vi "Analisis de fotos con video al tiempo.vi"() -> ()   [LabVIEW 2017]
uses:
  <vilib>/userdefined/High Color/IMAQdx.ctl
  <vilib>/vision/driver/NI_Vision_Acquisition_Software.lvlib
panel:
  in  "Puerto camara":T1
  in  "stop":bool
  out "Video":T2(plugin-control)
  in  "OK Button":bool
  out "Reconocimiento 2":T2(plugin-control)
  out "String (OCR/OCV 2\n)":string
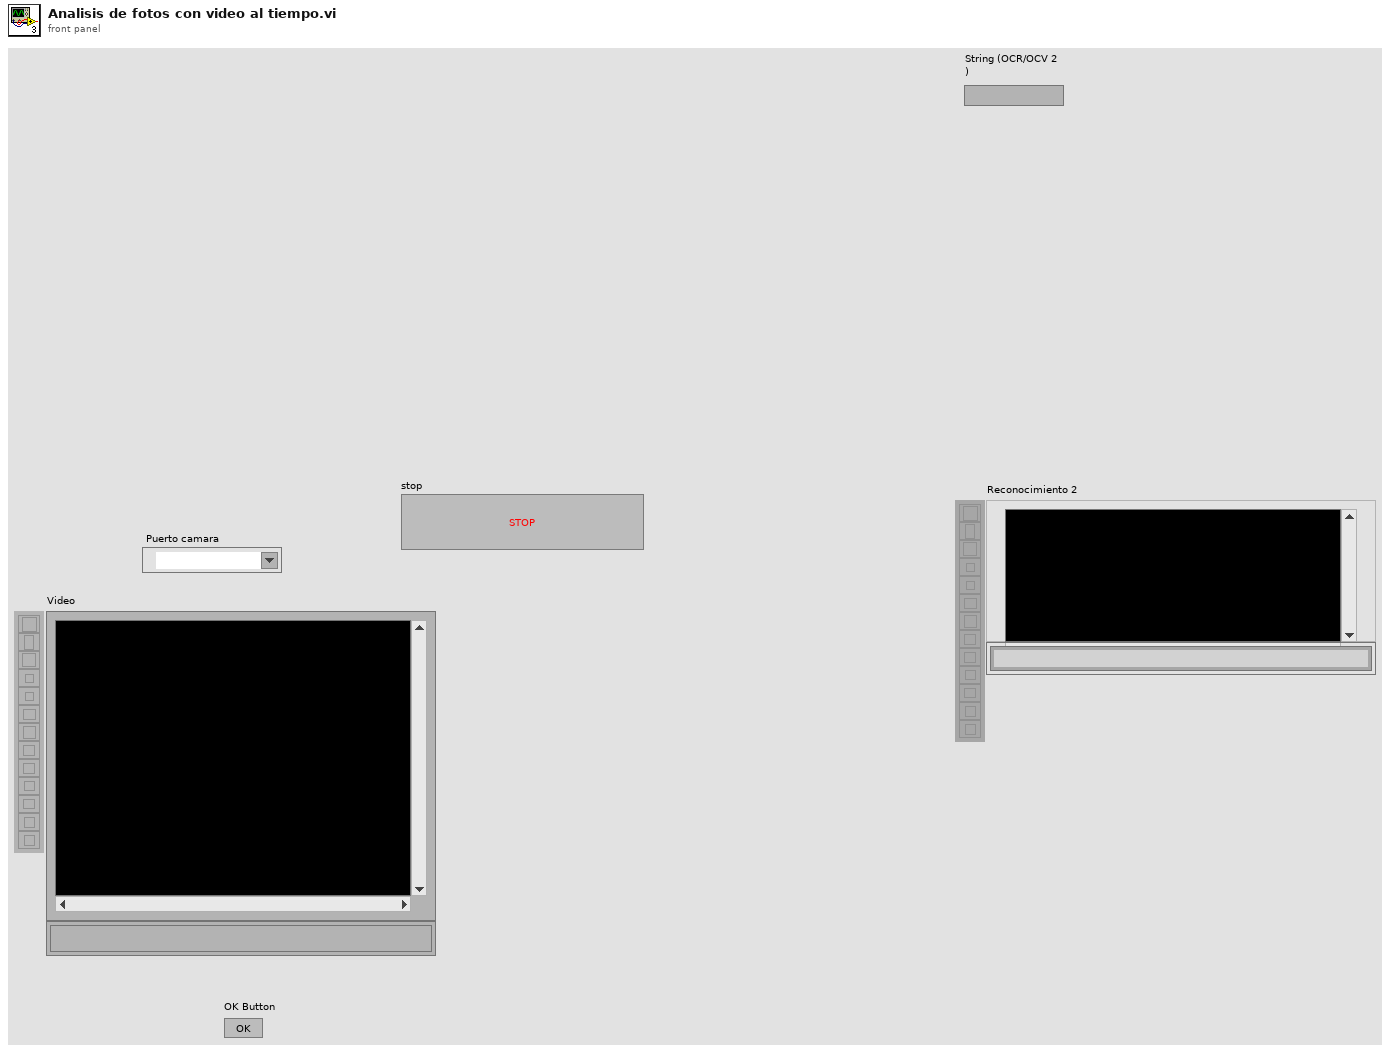
[diagram p1: front panel]
types:
  T1 = typedef "IMAQdx.ctl" = refnum<k21>
  T2 = typedef "IMAQ Image.ctl" = refnum<image>
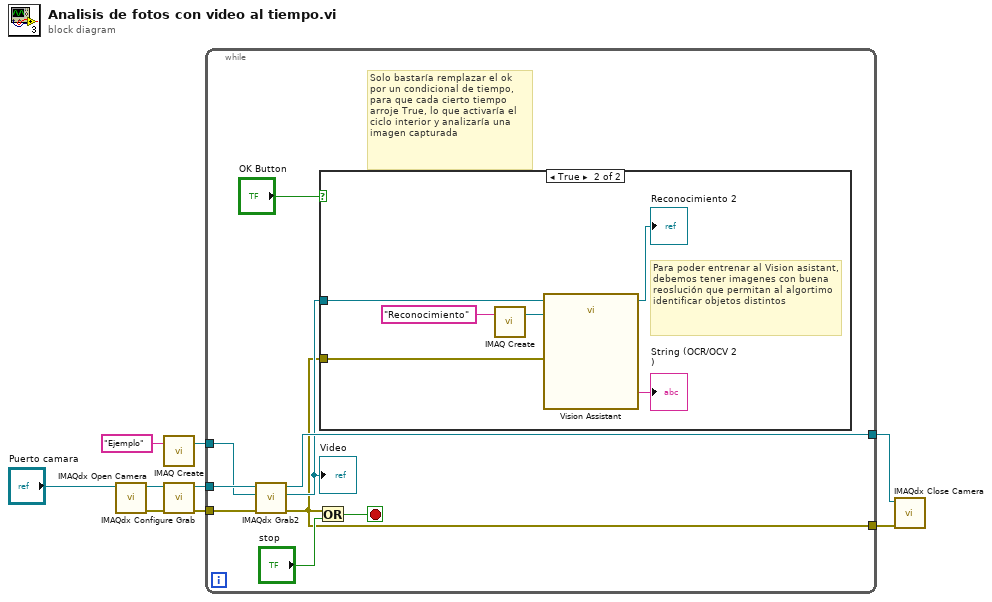
[diagram p0: block diagram]
diagram:
  n1 = call <vilib>:"IMAQdx Open Camera.vi"("Session In"="Puerto camara") -> ("error out"=w4:errorcluster, "Session Out"=w5:T1)  [unwired: 9 in]
  n2 = call "IMAQ Create"("Image Name"="Ejemplo") -> ("New Image"=w1:T2)  [unwired: 4 in, 1 out]
  n3 = call <vilib>:"IMAQdx Configure Grab.vi"("error in"=w4, "Session In"=w5) -> ("error out"=w3:errorcluster, "Session Out"=w6:T1)  [unwired: 8 in]
  n4 = while {
    tunnel: [w18] -> w7
    tunnel: w6 -> [w17]
    tunnel: w3 -> [w16]
    tunnel: [w11] -> w2
    tunnel: w1 -> [w15]
    stop <- w13 stop-if-true
    # "Solo bastaría remplazar el ok por un condicional de tiempo, para que cada cierto tiempo arroje True, lo que activaría el  ciclo interior y analizaría una imagen capturada"
    n5 = call <vilib>:"IMAQdx Grab2.vi"("error in"=w16, "Image In"=w15, "Session In"=w17) -> ("error out"=w11:errorcluster, "Image Out"=w12:T2, "Session Out"=w18:T1)  [unwired: 5 in, 1 out]
    "Video" <- w12
    n6 = Or(x=w11, y="stop") -> (x .or. y?=w13:bool)
    n7 = case shown="True" "OK Button" {
      tunnel: w12 -> [_ w20]
      tunnel: w11 -> [_ w19]
      frame False {
      }
      frame True {
        # "Para poder entrenar al Vision asistant, debemos tener imagenes con buena reoslución que permitan al algortimo identificar objetos distintos"
        n8 = call "IMAQ Create"("Image Name"="Reconocimiento") -> ("New Image"=w22:T2)  [unwired: 4 in, 1 out]
        n9 = call "Vision Assistant"("Image In"=w20, "Image Dst"=w22, "error in"=w19) -> ("Image Out"=→"Reconocimiento 2":T2, "String (OCR/OCV 3)"=→"String (OCR/OCV 2\n)":string)  [unwired: 22 in, 1 out]
      }
    }
  }
  n10 = call <vilib>:"IMAQdx Close Camera.vi"("error in"=w2, "Session In"=w7) -> ()  [unwired: 9 in, 1 out]
